vi "M07 Energy storage.vi"(11 "NXT/EV3":T1) -> (3 "EV3 out":T1)   [LabVIEW 2016]
uses:
  <vilib>/NXT/Subs/LVHSConnector.ctl
  <vilib>/NXT/LegoClasses/BrickReference/BrickReference.lvclass
  <vilib>/NXT/Block Support/NXT_InputPort.ctl
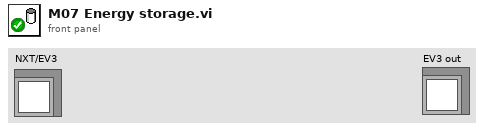
[diagram p1: front panel]
types:
  T1 = typedef "LVHSConnector.ctl" = refnum<class "BrickReference.lvclass">
  T2 = typedef "NXT_InputPort.ctl" = u32
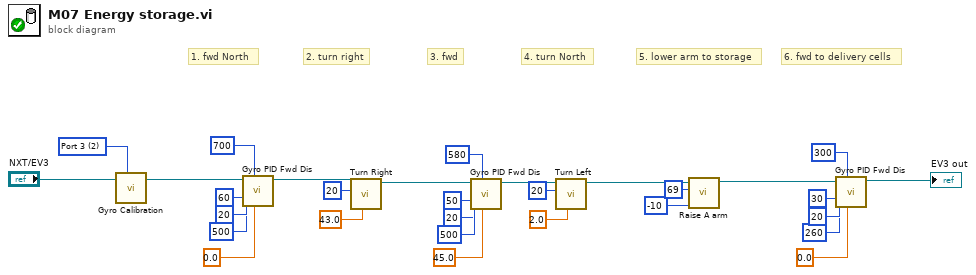
[diagram p0: block diagram]
diagram:
  w24 = T2 2 items=["Port 1", "Port 2", "Port 3", "Port 4"] ("Port (Port 1)")
  # "6. fwd to delivery cells"
  # "5. lower arm to storage"
  # "4. turn North"
  # "3. fwd"
  # "2. turn right"
  # "1. fwd North"
  n1 = call "Gyro Calibration.vi"("Port (Port 1)"=w24, "NXT/EV3"="NXT/EV3") -> ("NXT/EV3"=w25:T1)  [unwired: 5 in, 2 out]
  n2 = call "Gyro PID Fwd Dis.vi"("Target angle"=sgl 0.0, "Threshold to stop"=700, "Threshold to slow"=500, "Min. speed"=20, "Max. speed"=60, "EV3 in"=w25) -> ("EV3 out"=w22:T1)  [unwired: 5 in]
  n3 = call "Turn Right.vi"("Turning angle"=sgl 43.0, "Motor B (right)"=i8 20, "EV3 in"=w22) -> ("EV3 out"=w14:T1)  [unwired: 8 in]
  n4 = call "Gyro PID Fwd Dis.vi"("Target angle"=sgl 45.0, "Threshold to stop"=580, "Threshold to slow"=500, "Min. speed"=20, "Max. speed"=50, "EV3 in"=w14) -> ("EV3 out"=w13:T1)  [unwired: 5 in]
  n5 = call "Turn Left.vi"("Turning angle"=sgl 2.0, "Motor B (right)"=i8 20, "EV3 in"=w13) -> ("EV3 out"=w8:T1)  [unwired: 8 in]
  n6 = call "Raise A arm.vi"("Power"=i8 -10, "Rotation"=69, "EV3 in"=w8) -> ("EV3 out"=w2:T1)  [unwired: 8 in]
  n7 = call "Gyro PID Fwd Dis.vi"("Target angle"=sgl 0.0, "Threshold to stop"=300, "Threshold to slow"=260, "Min. speed"=20, "Max. speed"=30, "EV3 in"=w2) -> ("EV3 out"=→"EV3 out":T1)  [unwired: 5 in]
